vi "Create Path (segments).vi"(5 "URI-Component.Path":refnum<class "URI-Component.Path.lvclass">, 8 "error in (no error)":errorcluster, 11 "Segments":string[](array[string])) -> (0 "error out":errorcluster, 2 "Path type":T1=enum."path-abempty", 3 "URI-Component.Path":refnum<class "URI-Component.Path.lvclass">)   [LabVIEW 2013, in "openURI.lvlib" / "URI-Component.Path.lvclass"]
uses:
  URI-Component.Path.lvclass
  path type -- enum.ctl
  URI-Component.Path.lvclass/URI-Component.Path.ctl
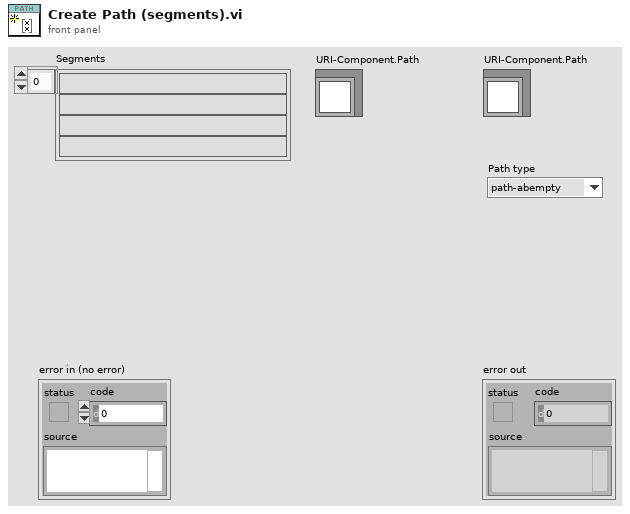
[diagram p1: front panel]
types:
  T1 = typedef "openURI.lvlib/URI-Component.Path.lvclass/path type -- enum.ctl" = enum16{"invalid", "path-abempty", "path-absolute", "path-noscheme", "path-rootless", "path-empty"}
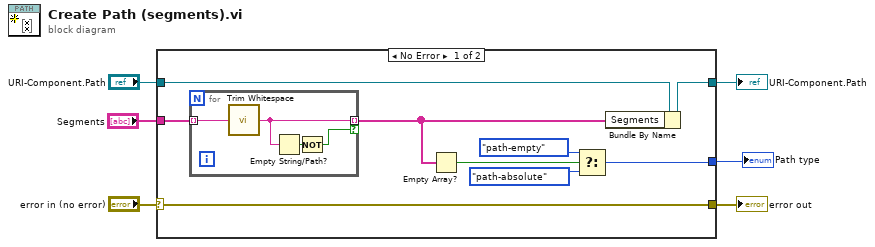
[diagram p0: block diagram]
diagram:
  n1 = case shown="No Error" "error in (no error)" {
    selector: "error in (no error)" -> [w15 w21]
    tunnel: [w15 w21] -> w5
    tunnel: [w13 w20] -> w3
    tunnel: "URI-Component.Path" -> [w14 w20]
    tunnel: "Segments" -> [w8 _]
    tunnel: [w9 _] -> w1
    frame No Error {
      n2 = for {
        tunnel: w8 -> [w19] mode=indexing
        tunnel: [w18] -> w7 mode=indexing if=w16
        n3 = call <vilib>:"Trim Whitespace.vi"("string"=w19) -> ("trimmed string"=w18:string)  [unwired: 1 in]
        n4 = Empty String/Path?(string/path=w18) -> (empty?=w17:bool)
        n5 = Not(x=w17) -> (.not. x?=w16:bool)
      }
      n6 = Empty Array?(array=w7) -> (empty?=w12:bool)
      n7 = Select(t=path_type_--_enum."path-empty" ("Path type"), s=w12, f=path_type_--_enum."path-absolute" ("Path type")) -> (s? t:f=w9:T1)
      n8 = Bundle By Name(cluster=w14, "Segments"=w7) -> (w13:refnum<class "URI-Component.Path.lvclass">)
    }
    frame Error {
    }
  }
  "error out" <- w5
  "URI-Component.Path" <- w3
  "Path type" <- w1
